vi "NATS Client Publish.vi"(8 "error in":errorcluster, 9 "payload":string, 10 "subject":string, 11 "NATS Client.lvlib:NATS Client.lvclass":refnum<class "NATS Client.lvclass">) -> (0 "error out":errorcluster)   [LabVIEW 2024, in "NATS Client.lvlib" / "NATS Client.lvclass"]
uses:
  NATS Client.lvclass
  NATS Client.lvclass/NATS Client.ctl
  NATS Core.lvlib
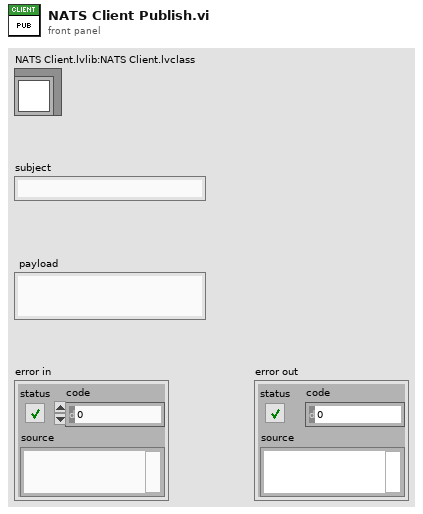
[diagram p1: front panel]
types:
  T1 = typedef "NATS Core.lvlib/nats connection.ctl" = cluster{"connection ID":refnum<k5>, "server INFO":string, "timeout ms":i32, "verbose?":bool, "server headers?":bool, "client headers?":bool}
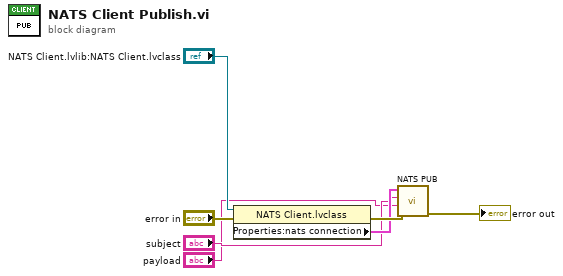
[diagram p0: block diagram]
diagram:
  n1 = property class="NATS Client.lvclass"(reference="NATS Client.lvlib:NATS Client.lvclass", error in="error in") -> (error out=w7:errorcluster, "Properties:nats connection"=w3:T1)  [unwired: 1 out]
  n2 = call "NATS PUB.vi"("error in"=w7, "payload"="payload", "subject"="subject", "nats connection in"=w3) -> ("error out"=→"error out":errorcluster)  [unwired: 6 in, 1 out]
